vi "Bundle Script_In Place_Mark disabled items.vi"(10 "Displayed Items":T1[](array[typedef]), 11 "Cluster Items":T1[](array[typedef])) -> (3 "Dialog Items":T1[](array[typedef]))   [LabVIEW 2023]
doc: "Inplace clsuter bundlers don't allow multiple elements of the same data value, so here we set to disable those items that are already in the bundlers."
uses:
  Cluster Element Description.ctl
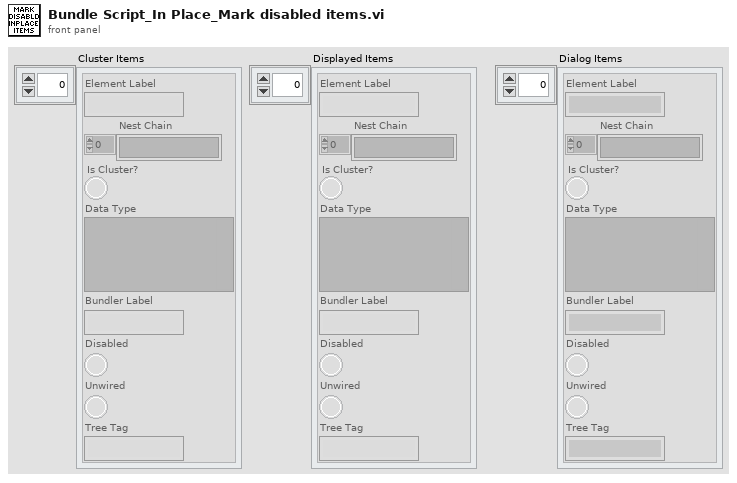
[diagram p1: front panel]
types:
  T1 = typedef "Cluster Element Description.ctl" = cluster{"Element Label":string, "Nest Chain":string[], "Is Cluster?":bool, "Data Type":variant, "Bundler Label":string, "Disabled":bool, "Unwired":bool, "Tree Tag":string}
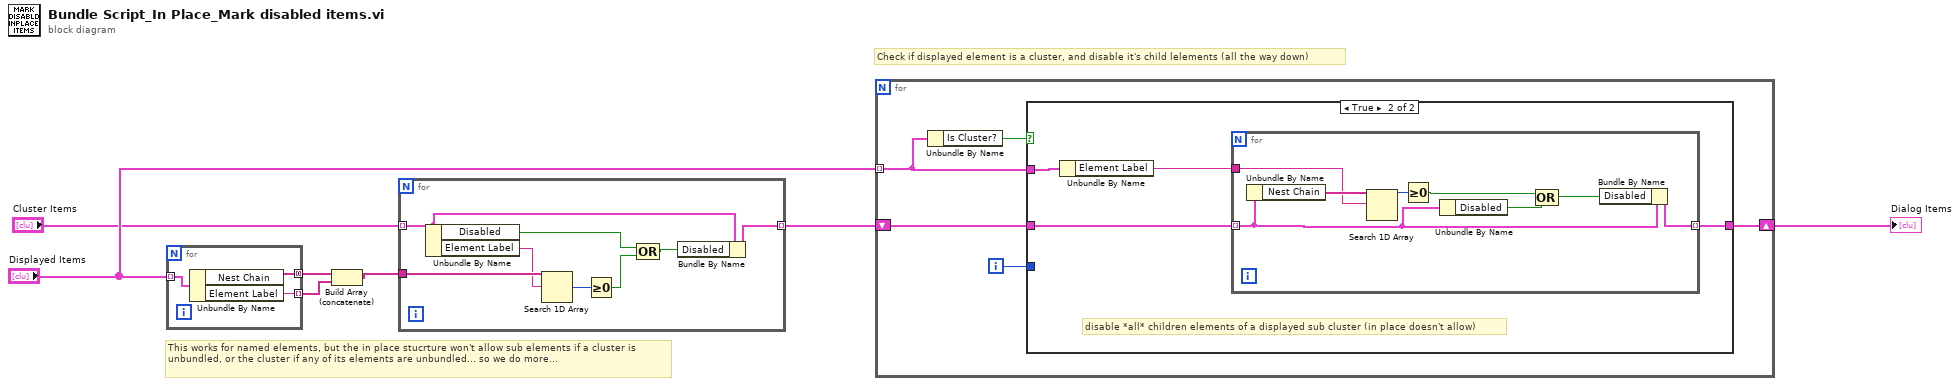
[diagram p0: block diagram]
diagram:
  # "This works for named elements, but the in place stucrture won't allow sub elements if a cluster is unbundled, or the cluster if any of its elements are unbundled... so we do more..."
  # "Check if displayed element is a cluster, and disable it's child lelements (all the way down)"
  n1 = for {
    tunnel: "Displayed Items" -> [w10] mode=indexing
    tunnel: [w9] -> w3 mode=concatenating
    tunnel: [w8] -> w2 mode=indexing
    n2 = Unbundle By Name(w10) -> ("Nest Chain"=w9:string[], "Element Label"=w8:string)
  }
  n3 = Build Array (concatenate)(w3, w2) -> (w1:string[])
  n4 = for {
    tunnel: "Cluster Items" -> [w15] mode=indexing
    tunnel: w1 -> [w18]
    tunnel: [w16] -> w4 mode=indexing
    n5 = Unbundle By Name(w15) -> ("Disabled"=w13:bool, "Element Label"=w14:string)
    n6 = Search 1D Array(1D array=w18, element=w14) -> (index of element=w17:i32)  [unwired: 1 in]
    n7 = Greater Or Equal To 0?(x=w17) -> (x >= 0?=w12:bool)
    n8 = Compound Arithmetic op=OR(w13, w12) -> (w11:bool)
    n9 = Bundle By Name(cluster=w15, "Disabled"=w11) -> (w16:T1)
  }
  n10 = for {
    tunnel: "Displayed Items" -> [w22] mode=indexing
    shift-right: [w19] -> w6
    shift-left: w4 -> [w20]
    i -> [w21]
    n11 = Unbundle By Name(w22) -> ("Is Cluster?"=w23:bool)
    n12 = case shown="True" w23 {
      tunnel: w22 -> [_ w28]
      tunnel: w21 -> [_ _]
      tunnel: w20 -> [w24 w27]
      tunnel: [w24 w25] -> w19
      frame False {
      }
      frame True {
        # "disable *all* children elements of a displayed sub cluster (in place doesn't allow)"
        n13 = Unbundle By Name(w28) -> ("Element Label"=w26:string)
        n14 = for {
          tunnel: w27 -> [w35] mode=indexing
          tunnel: w26 -> [w31]
          tunnel: [w36] -> w25 mode=indexing
          n15 = Unbundle By Name(w35) -> ("Nest Chain"=w32:string[])
          n16 = Search 1D Array(1D array=w32, element=w31) -> (index of element=w30:i32)  [unwired: 1 in]
          n17 = Greater Or Equal To 0?(x=w30) -> (x >= 0?=w29:bool)
          n18 = Unbundle By Name(w35) -> ("Disabled"=w34:bool)
          n19 = Compound Arithmetic op=OR(w29, w34) -> (w33:bool)
          n20 = Bundle By Name(cluster=w35, "Disabled"=w33) -> (w36:T1)
        }
      }
    }
  }
  "Dialog Items" <- w6
